vi "turning_handler.vi"(10 "dataCluster":T1, 11 "REST Client in":refnum<class "REST Client.lvclass">) -> (3 "REST Client out":refnum<class "REST Client.lvclass">)   [LabVIEW 2024]
uses:
  <vilib>/addons/_JKI.lib/REST Client/classes/REST Client/REST Client.lvclass
  typeDef/dataCluster.ctl
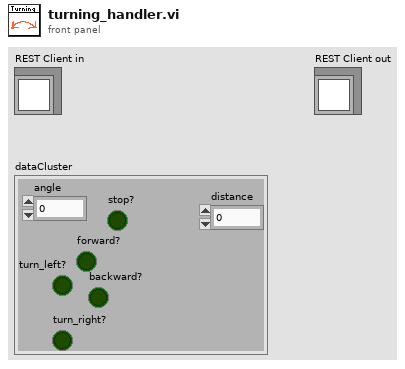
[diagram p1: front panel]
types:
  T1 = typedef "dataCluster.ctl" = cluster{"angle":dbl, "turn_left?":bool, "turn_right?":bool, "forward?":bool, "backward?":bool, "stop?":bool, "distance":dbl}
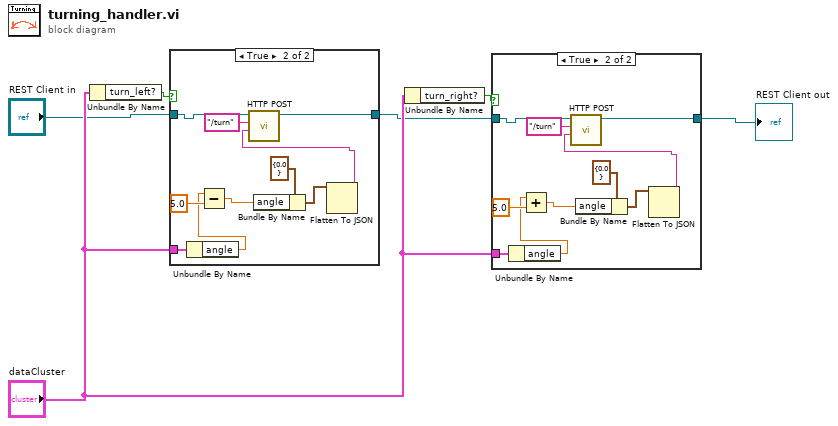
[diagram p0: block diagram]
diagram:
  n1 = Unbundle By Name("dataCluster") -> ("turn_left?"=w1:bool)
  n2 = case shown="True" w1 {
    tunnel: "REST Client in" -> [w7 w11]
    tunnel: [w7 w9] -> w3
    tunnel: "dataCluster" -> [_ w10]
    frame False {
    }
    frame True {
      n3 = Unbundle By Name(w10) -> ("angle"=w12:dbl)
      n4 = Subtract(x=w12, y=5.0) -> (x-y=w14:dbl)
      n5 = Bundle By Name(cluster=cluster{"angle":dbl} {"angle"=0.0}, "angle"=w14) -> (w16:cluster{"angle":dbl})
      n6 = Flatten To JSON(anything=w16) -> (JSON string=w8:string)  [unwired: 2 in, 1 out]
      n7 = call-dynamic "HTTP POST.vi"("Request body"=w8, "Path"="/turn", "REST Client in"=w11) -> ("REST Client out"=w9:refnum<class "REST Client.lvclass">)  [unwired: 3 in, 5 out]
    }
  }
  n8 = Unbundle By Name("dataCluster") -> ("turn_right?"=w6:bool)
  n9 = case shown="True" w6 {
    tunnel: w3 -> [w18 w22]
    tunnel: [w18 w20] -> w4
    tunnel: "dataCluster" -> [_ w21]
    frame False {
    }
    frame True {
      n10 = Unbundle By Name(w21) -> ("angle"=w23:dbl)
      n11 = Add(x=w23, y=5.0) -> (x+y=w25:dbl)
      n12 = Bundle By Name(cluster=cluster{"angle":dbl} {"angle"=0.0}, "angle"=w25) -> (w27:cluster{"angle":dbl})
      n13 = Flatten To JSON(anything=w27) -> (JSON string=w19:string)  [unwired: 2 in, 1 out]
      n14 = call-dynamic "HTTP POST.vi"("Request body"=w19, "Path"="/turn", "REST Client in"=w22) -> ("REST Client out"=w20:refnum<class "REST Client.lvclass">)  [unwired: 3 in, 5 out]
    }
  }
  "REST Client out" <- w4
